vi "Task Panel Closed.vi"(8 "error in (no error)":errorcluster, 11 "GUI in":refnum<class "GUI.lvclass">) -> (0 "error out":errorcluster, 3 "GUI out":refnum<class "GUI.lvclass">)   [LabVIEW 2020, in "GUI.lvlib" / "GUI.lvclass"]
uses:
  GUI.lvclass
  C:/Program Files/National Instruments/LabVIEW 2020/vi.lib/ActorFramework/Actor/Actor.lvclass
  GUI.lvclass/GUI.ctl
  <vilib>/ActorFramework/Actor/Actor.lvclass/Actor.ctl
  <vilib>/ActorFramework/Message Enqueuer/Message Enqueuer.lvclass/Message Enqueuer.ctl
  GUI Interface Messages/End Preview Msg/End Preview Msg.lvclass/End Preview Msg.ctl
  <vilib>/ActorFramework/Message Enqueuer/Init from Existing Queue.vi
  <vilib>/ActorFramework/Message Enqueuer/Enqueue.vi
  GUI Interface Messages/End Preview Msg/End Preview Msg.lvclass
  C:/Program Files/National Instruments/LabVIEW 2020/vi.lib/ActorFramework/Message/Message.lvclass
  <vilib>/ActorFramework/Message Priority Queue/Priority Enqueue.vi
  <vilib>/ActorFramework/Message Enqueuer/Message Enqueuer.lvclass
  <vilib>/ActorFramework/Actor/Actor.lvclass
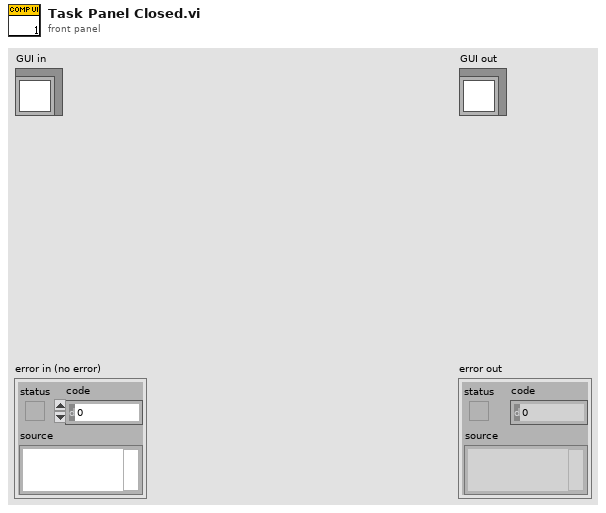
[diagram p1: front panel]
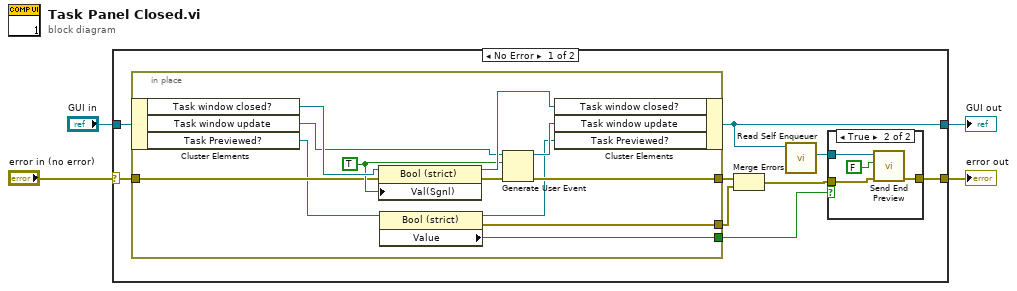
[diagram p0: block diagram]
diagram:
  n1 = case shown="No Error" "error in (no error)" {
    selector: "error in (no error)" -> [w12 w32]
    tunnel: [w9 w32] -> w3
    tunnel: [w11 w31] -> w1
    tunnel: "GUI in" -> [w13 w31]
    frame No Error {
      n2 = in-place {
        in-place-border: w12 -> [w26]
        in-place-border: [w23] -> w7
        in-place-border: [w21] -> w8
        in-place-border: [w19] -> w6
        w27 = TRUE ("Value (Signaling)")
        n3 = in-place-cluster #1(w13) -> ("Task window closed?"=w30:refnum<vi>, "Task window update"=w28:refnum<user-event>, "Task Previewed?"=w22:refnum<vi>)
        n4 = property class="Bool (strict)"(reference=w30, error in=w26, "Val(Sgnl)"=w27) -> (reference out=w29:refnum<vi>, error out=w25:errorcluster)
        n5 = property class="Bool (strict)"(reference=w22) -> (reference out=w20:refnum<vi>, error out=w21:errorcluster, "Value"=w19:bool)  [unwired: 1 in]
        n6 = Generate User Event(user event=w28, event data cluster=w27, error in=w25) -> (user event out=w24:refnum<user-event>, error out=w23:errorcluster)  [unwired: 1 in]
        n7 = in-place-cluster #1("Task window closed?"=w29, "Task window update"=w24, "Task Previewed?"=w20) -> (w11:refnum<class "GUI.lvclass">)
      }
      n8 = Merge Errors(w7, w8) -> (w5:errorcluster)
      n9 = call <vilib>:"Read Self Enqueuer.vi"("Actor"=w11) -> ("Self Enqueuer"=w10:refnum<class "Message Enqueuer.lvclass">)  [unwired: 10 in]
      n10 = case shown="True" w6 {
        tunnel: w10 -> [_ w18]
        tunnel: [w14 w16] -> w9
        tunnel: w5 -> [w14 w15]
        frame False {
        }
        frame True {
          n11 = call "Send End Preview.vi"("error in (no error)"=w15, "Preview"=FALSE, "Message Enqueuer"=w18) -> ("error out"=w16:errorcluster)  [unwired: 7 in, 1 out]
        }
      }
    }
    frame Error {
    }
  }
  "error out" <- w3
  "GUI out" <- w1
